vi "getStageFromXmlNative.vi"(8 "error in (no error)":errorcluster, 10 "eventXML":refnum<k20>, 11 "ScriptEvent in":refnum<class "ScriptEvent.lvclass">) -> (0 "error out":errorcluster, 2 "eventXML out":refnum<k20>, 3 "ScriptEvent out":refnum<class "ScriptEvent.lvclass">)   [LabVIEW 2009, in "Tools.lvlib" / "Scripting.lvlib" / "ScriptEvent.lvclass"]
uses:
  ScriptEvent.lvclass
  <vilib>/xml/Close Reference(Node).vi
  <vilib>/xml/NI_XML.lvlib
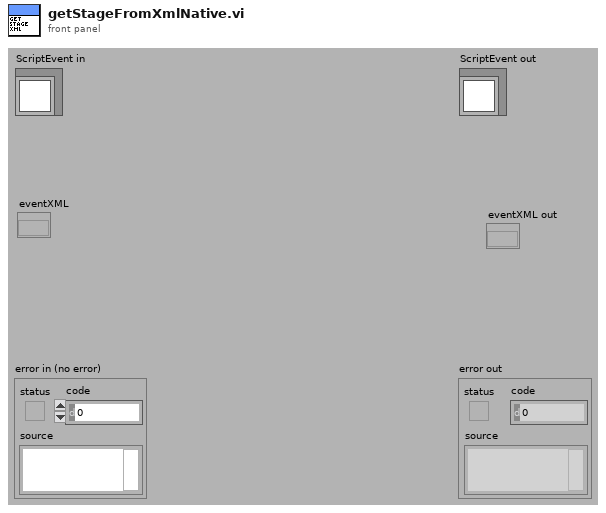
[diagram p1: front panel]
types:
  T1 = enum16{"Initialise", "MOT", "Molasses", "Optical Pumping", "Magnetic Trap", "RF Cooling", "Manipulation", "Switch Off", "Absorption Imaging", "Fluorscence Imaging", "Shut Down"}
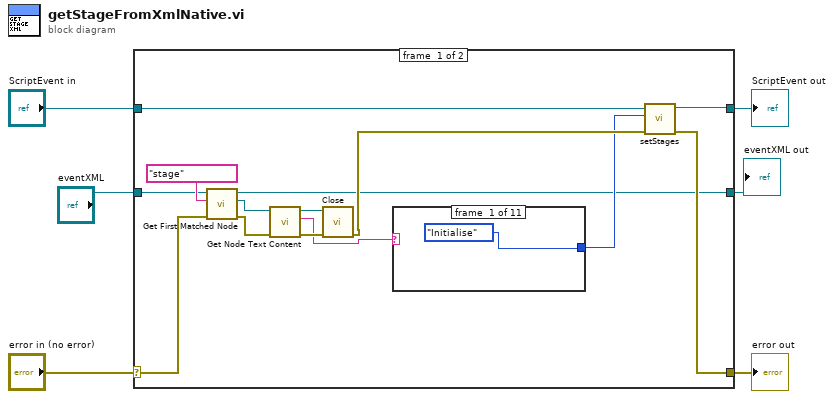
[diagram p0: block diagram]
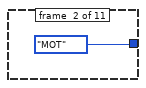
[diagram p2: hidden frame]
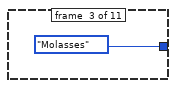
[diagram p3: hidden frame]
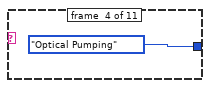
[diagram p4: hidden frame]
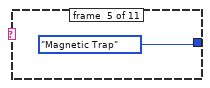
[diagram p5: hidden frame]
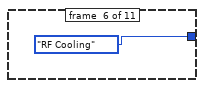
[diagram p6: hidden frame]
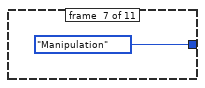
[diagram p7: hidden frame]
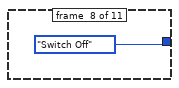
[diagram p8: hidden frame]
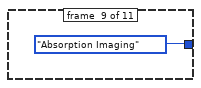
[diagram p9: hidden frame]
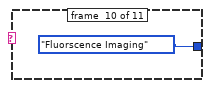
[diagram p10: hidden frame]
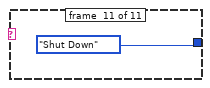
[diagram p11: hidden frame]
diagram:
  n1 = case shown="No Error" "error in (no error)" {
    selector: "error in (no error)" -> [w8 w33]
    tunnel: [w9 w33] -> w5
    tunnel: [w13 w32] -> w3
    tunnel: "ScriptEvent in" -> [w12 w32]
    tunnel: "eventXML" -> [w15 _]
    tunnel: [w7 _] -> w1
    frame #0 {
      n2 = call <vilib>:"Get First Matched Node.vi"("error in (no error)"=w8, "XPath expression"="stage", "node in"=w15) -> ("error out"=w19:errorcluster, "node result"=w18:refnum<k20>, "node out"=w7:refnum<k20>)  [unwired: 6 in]
      n3 = call <vilib>:"Get Node Text Content.vi"("error in (no error)"=w19, "node in"=w18) -> ("error out"=w17:errorcluster, "node text"=w14:string, "node out"=w16:refnum<k20>)  [unwired: 7 in]
      n4 = call-poly <vilib>:"Close.vi"("error in (no error)"=w17, "node"=w16) -> ("error out"=w11:errorcluster)  [unwired: 7 in]
      n5 = case shown="\"Manipulation\"" w14 {
        tunnel: [T1."Initialise" ("Value") T1."MOT" ("Value") T1."Molasses" ("Value") T1."Optical Pumping" ("Value") T1."Magnetic Trap" ("Value") T1."RF Cooling" ("Value") T1."Manipulation" ("Value") T1."Switch Off" ("Value") T1."Absorption Imaging" ("Value") T1."Fluorscence Imaging" ("Value") T1."Shut Down" ("Value")] -> w10
        frame #0 {
        }
        frame #1 {
        }
        frame #2 {
        }
        frame #3 {
        }
        frame #4 {
        }
        frame #5 {
        }
        frame #6 {
        }
        frame #7 {
        }
        frame #8 {
        }
        frame #9 {
        }
        frame #10 {
        }
      }
      n6 = call-dynamic "setStages.vi"("error in (no error)"=w11, "Stage"=w10, "ScriptEvent.lvclass in"=w12) -> ("error out"=w9:errorcluster, "ScriptEvent.lvclass out"=w13:refnum<class "ScriptEvent.lvclass">)  [unwired: 7 in]
    }
    frame #1 {
    }
  }
  "error out" <- w5
  "ScriptEvent out" <- w3
  "eventXML out" <- w1
